vi "MS5607_GetRawPressure.vi"(8 "error in (no error)":errorcluster, 10 "OSR":enum8{"256", "512", "1024", "2048"}(ring)=enum."2048", 11 "Slave Address (7-bit)":u8) -> (0 "error out":errorcluster, 3 "Raw Pressure Data":u32)   [LabVIEW 2016]
uses:
  <vilib>/myRIO/Instrument Drivers/Onboard IO/I2C/vis/Configure.vi
  <vilib>/myRIO/Instrument Drivers/Onboard IO/I2C/vis/Write.vi
  <vilib>/myRIO/Instrument Drivers/Onboard IO/I2C/vis/Read.vi
  <vilib>/myRIO/Instrument Drivers/Onboard IO/I2C/vis/Smart Open.vi
  <vilib>/Utility/error.llb/Error Cluster From Error Code.vi
  <vilib>/myRIO/Common/Instrument Driver Framework/myRIO v1.0/I2C/vis/myRIO v1.0 Configure I2C.vi
  <vilib>/myRIO/Common/Instrument Driver Framework/myRIO v1.0/I2C/vis/myRIO v1.0 Write I2C.vi
  <vilib>/myRIO/Common/Instrument Driver Framework/myRIO v1.0/I2C/vis/myRIO v1.0 Read I2C.vi
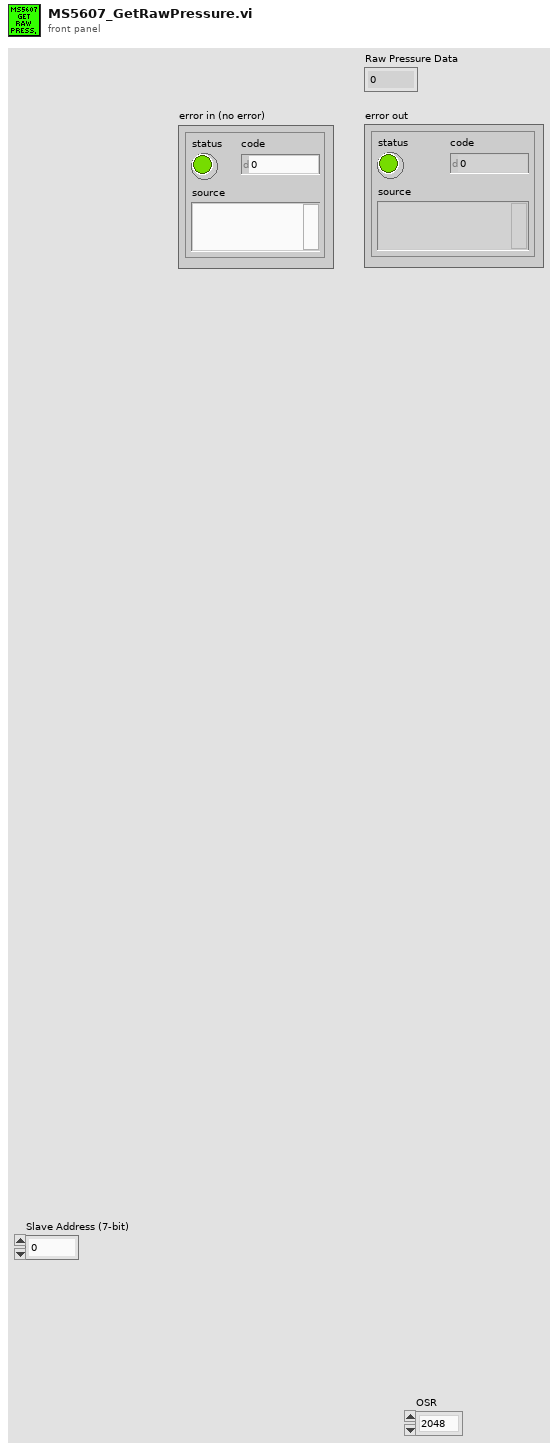
[diagram p1: front panel]
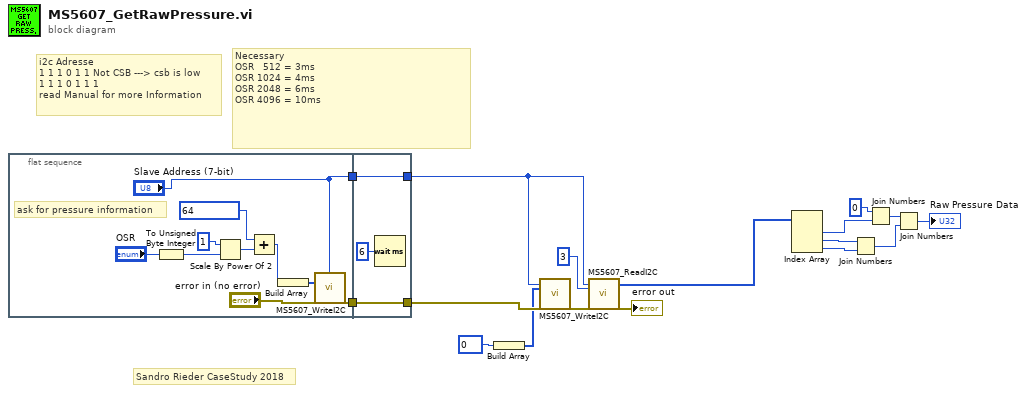
[diagram p0: block diagram]
diagram:
  # "Sandro Rieder CaseStudy 2018"
  # "Necessary\nOSR   512 = 3ms\nOSR 1024 = 4ms\nOSR 2048 = 6ms\nOSR 4096 = 10ms"
  # "i2c Adresse\n1 1 1 0 1 1 Not CSB ---> csb is low\n1 1 1 0 1 1 1\nread Manual for more Information"
  n1 = flat-sequence {
    tunnel: ["Slave Address (7-bit)"] -> w3
    tunnel: [w19] -> w2
    tunnel: [w29] -> w6
    tunnel: [w30] -> w7
    tunnel: w3 -> [w30]
    tunnel: w2 -> [w29]
    frame #0 {
      # "ask for pressure information"
      n2 = To Unsigned Byte Integer(number="OSR") -> (unsigned 8bit integer=w22:u8)
      n3 = Scale By Power Of 2(n=u8 1, x=w22) -> (x*2^n=w23:u8)
      n4 = Add(x=u8 64, y=w23) -> (x+y=w24:u8)
      n5 = Build Array(w24) -> (w20:u8[])
      n6 = call "MS5607_WriteI2C.vi"("Slave Address (7-bit)"="Slave Address (7-bit)", "Bytes to Write"=w20, "error in (no error)"="error in (no error)") -> ("error out"=w19:errorcluster)  [unwired: 24 in]
    }
    frame #1 {
      n7 = Wait (ms)(milliseconds to wait=u32 6) -> ()  [unwired: 1 out]
    }
  }
  n8 = Build Array(u8 0) -> (w4:u8[])
  n9 = call "MS5607_WriteI2C.vi"("Slave Address (7-bit)"=w7, "Bytes to Write"=w4, "error in (no error)"=w6) -> ("error out"=w5:errorcluster)  [unwired: 24 in]
  n10 = call "MS5607_ReadI2C.vi"("Slave Address (7-bit)"=w7, "Byte Count"=u32 3, "error in (no error)"=w5) -> ("Bytes Read"=w9:u8[], "error out"=→"error out":errorcluster)  [unwired: 23 in]
  n11 = Index Array(array=w9) -> (element #1=w15:u8, element #2=w16:u8, element #3=w17:u8)  [unwired: 3 in]
  n12 = Join Numbers(hi=w16, lo=w17) -> ((hi.lo)=w12:u16)
  n13 = Join Numbers(hi=u8 0, lo=w15) -> ((hi.lo)=w13:u16)
  n14 = Join Numbers(hi=w13, lo=w12) -> ((hi.lo)=→"Raw Pressure Data":u32)
